vi "Encoder_Open4Encoders.vi"(0 "Rear Left Motor A":T6, 1 "Rear Left Motor B":T6, 2 "Rear Right Motor A":T6, 3 "Rear Right Motor B":T6, 4 "Front Left Motor A":T6, 5 "Front Left Motor B":T6, 6 "Front Right Motor A":T6, 7 "Front Right Motor B":T6, 8 "Front Right Motor Max":dbl, 10 "Front Left Motor Max":dbl, 12 "Rear Right Motor Max":dbl, 14 "Rear Left Motor Max":dbl) -> (21 "RobotEncoderRef Out":T5, 26 "error out":errorcluster)   [LabVIEW 2013]
uses:
  <vilib>/Rock Robotics/SystemInterfaces/DIO/FPGA_DIOChannel.ctl
  <vilib>/Rock Robotics/WPI/Encoder/WPI_EncoderDevRef.ctl
  <vilib>/Rock Robotics/SystemInterfaces/Encoder/FPGA_EncoderIdx.ctl
  <vilib>/Rock Robotics/SystemInterfaces/Counter/FPGA_CounterCtrSystemIndex.ctl
  <vilib>/Rock Robotics/WPI/Encoder/WPI_EncoderType.ctl
  <vilib>/Rock Robotics/WPI/Counter/WPI_CounterDigitalInputToDigitalSource.vi
panel:
  in  "error in (no error)":errorcluster
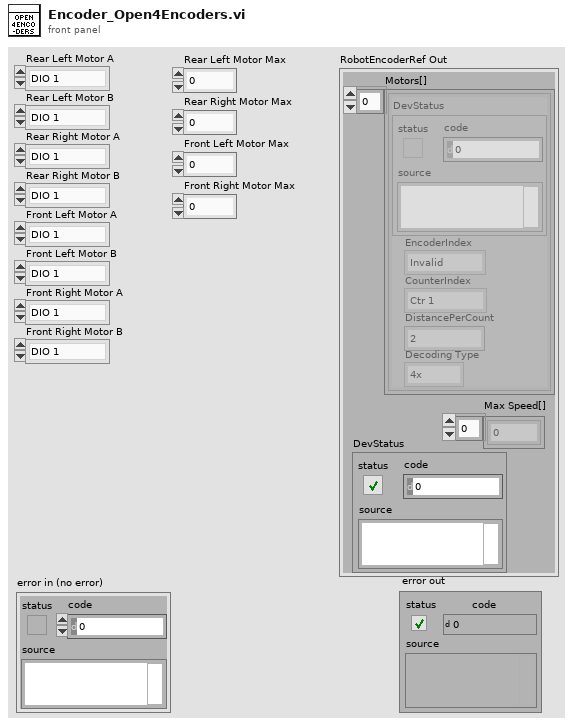
[diagram p1: front panel]
types:
  T1 = typedef "WPI_EncoderDevRef.ctl" = cluster{"DevStatus":errorcluster, "EncoderIndex":T2, "CounterIndex":T3, "DistancePerCount":dbl, "Decoding Type":T4}
  T2 = typedef "FPGA_EncoderIdx.ctl" = enum8{"Enc 0", "Enc 1", "Enc 2", "Enc 3", "Invalid"}
  T3 = typedef "FPGA_CounterCtrSystemIndex.ctl" = enum8{"Ctr 0", "Ctr 1", "Ctr 2", "Ctr 3", "Ctr 4", "Ctr 5", "Ctr 6", "Ctr 7", "Invalid"}
  T4 = typedef "WPI_EncoderType.ctl" = enum16{"1x", "2x", "4x"}
  T5 = cluster{"Motors[]":T1[], "DevStatus":errorcluster, "Max Speed[]":dbl[]}
  T6 = typedef "FPGA_DIOChannel.ctl" = enum8{"DIO 1", "DIO 2", "DIO 3", "DIO 4", "DIO 5", "DIO 6", "DIO 7", "DIO 8", "DIO 9", "DIO 10", "DIO 11", "DIO 12", "DIO 13", "DIO 14", "Invalid"}
  T7 = typedef "WPI_DigitalInputDevRef.ctl" = cluster{"DevStatus":errorcluster, "DIO Channel":T6, "Digital Module":T8}
  T8 = typedef "FPGA_TypedefDigitalModule.ctl" = enum16{"Digital Module 1", "Digital Module 2"}
  T9 = typedef "FPGA_CounterEncoderSourceConvertionLVSourceType.ctl" = cluster{"DevStatus":errorcluster, "AnalogTriggerMode?":bool, "DigitalMode":cluster{"Digital Module":T8, "DIO Channel":T10}, "AnalogTriggerMode":cluster{"AnalogTriggerIndex":T11, "OutputType":T12}}
  T10 = typedef "FPGA_DIODigitalSourceChannel.ctl" = enum8{"DIO 1", "DIO 2", "DIO 3", "DIO 4", "DIO 5", "DIO 6", "DIO 7", "DIO 8", "DIO 9", "DIO 10", "DIO 11", "DIO 12", "DIO 13", "DIO 14", "Disabled"}
  T11 = typedef "FPGA_AnalogTriggerIndex.ctl" = enum8{"Trig 0", "Trig 1", "Trig 2", "Trig 3", "Trig 4", "Trig 5", "Trig 6", "Trig 7", "Invalid"}
  T12 = typedef "FPGA_AnalogTriggerOutType.ctl" = enum16{"InWindow", "TriggerState", "Rising", "Falling"}
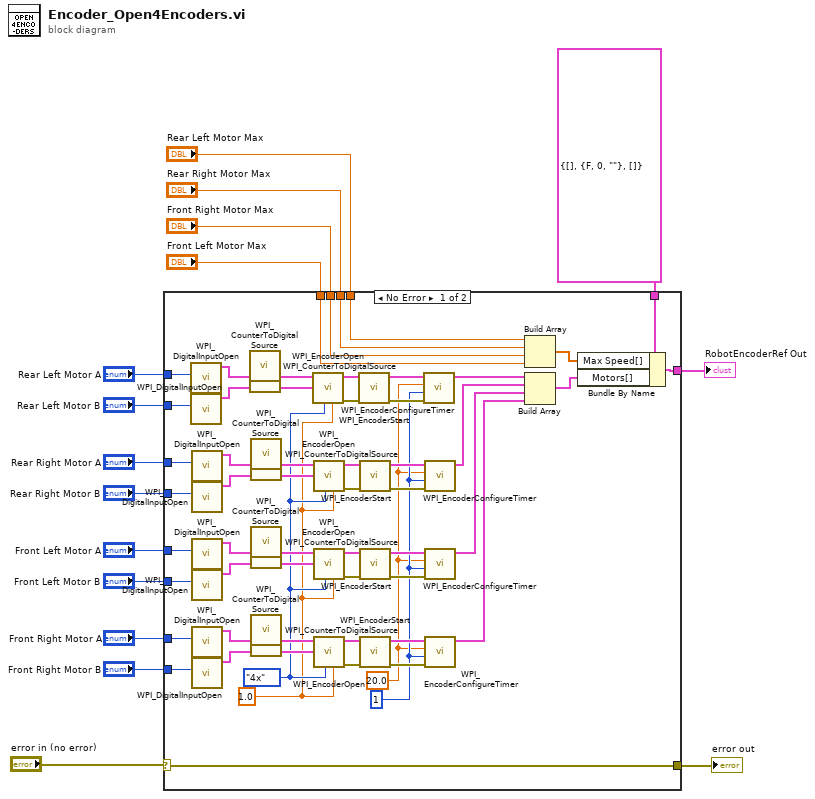
[diagram p0: block diagram]
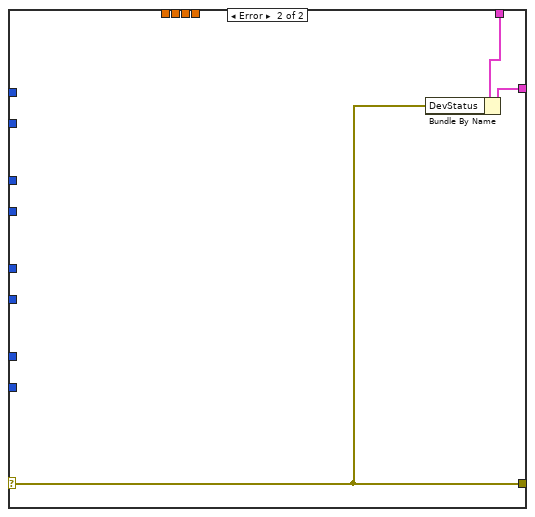
[diagram p2: hidden frame]
diagram:
  n1 = case shown="No Error" "error in (no error)" {
    selector: "error in (no error)" -> [w23 w74]
    tunnel: "Rear Left Motor A" -> [w37 _]
    tunnel: "Rear Left Motor B" -> [w36 _]
    tunnel: "Rear Right Motor A" -> [w35 _]
    tunnel: "Rear Right Motor B" -> [w34 _]
    tunnel: "Front Left Motor A" -> [w33 _]
    tunnel: "Front Left Motor B" -> [w32 _]
    tunnel: "Front Right Motor A" -> [w31 _]
    tunnel: "Front Right Motor B" -> [w30 _]
    tunnel: [w25 w75] -> w7
    tunnel: T5 {"Motors[]"=[], "DevStatus"={"status"=FALSE, "code"=0, "source"=""}, "Max Speed[]"=[]} ("RobotEncoderRef Out") -> [w24 w76]
    tunnel: [w23 w74] -> w8
    tunnel: "Front Left Motor Max" -> [w20 _]
    tunnel: "Front Right Motor Max" -> [w21 _]
    tunnel: "Rear Right Motor Max" -> [w19 _]
    tunnel: "Rear Left Motor Max" -> [w18 _]
    frame No Error {
      w27 = u8 1 ("Number Samples to Average")
      w26 = 20.0 ("Minimum Rate")
      w28 = 1.0 ("DistancePerCount")
      w29 = WPI_EncoderType."4x" ("Decoding Type")
      n2 = call <vilib>:"WPI_DigitalInputOpen.vi"("DIO Channel"=w37) -> ("DigitalInputDevRef"=w66:T7)  [unwired: 9 in, 1 out]
      n3 = call <vilib>:"WPI_DigitalInputOpen.vi"("DIO Channel"=w36) -> ("DigitalInputDevRef"=w67:T7)  [unwired: 9 in, 1 out]
      n4 = call <vilib>:"WPI_DigitalInputOpen.vi"("DIO Channel"=w35) -> ("DigitalInputDevRef"=w58:T7)  [unwired: 9 in, 1 out]
      n5 = call <vilib>:"WPI_DigitalInputOpen.vi"("DIO Channel"=w34) -> ("DigitalInputDevRef"=w59:T7)  [unwired: 9 in, 1 out]
      n6 = call <vilib>:"WPI_DigitalInputOpen.vi"("DIO Channel"=w33) -> ("DigitalInputDevRef"=w50:T7)  [unwired: 9 in, 1 out]
      n7 = call <vilib>:"WPI_DigitalInputOpen.vi"("DIO Channel"=w32) -> ("DigitalInputDevRef"=w51:T7)  [unwired: 9 in, 1 out]
      n8 = call <vilib>:"WPI_DigitalInputOpen.vi"("DIO Channel"=w31) -> ("DigitalInputDevRef"=w42:T7)  [unwired: 9 in, 1 out]
      n9 = call <vilib>:"WPI_DigitalInputOpen.vi"("DIO Channel"=w30) -> ("DigitalInputDevRef"=w43:T7)  [unwired: 9 in, 1 out]
      n10 = call-poly <vilib>:"WPI_CounterToDigitalSource.vi"("DigitalInputDevRef"=w66) -> ("Digital Source"=w69:T9)  [unwired: 6 in]
      n11 = call-poly <vilib>:"WPI_CounterToDigitalSource.vi"("DigitalInputDevRef"=w67) -> ("Digital Source"=w68:T9)  [unwired: 6 in]
      n12 = call-poly <vilib>:"WPI_CounterToDigitalSource.vi"("DigitalInputDevRef"=w58) -> ("Digital Source"=w61:T9)  [unwired: 6 in]
      n13 = call-poly <vilib>:"WPI_CounterToDigitalSource.vi"("DigitalInputDevRef"=w59) -> ("Digital Source"=w60:T9)  [unwired: 6 in]
      n14 = call-poly <vilib>:"WPI_CounterToDigitalSource.vi"("DigitalInputDevRef"=w50) -> ("Digital Source"=w53:T9)  [unwired: 6 in]
      n15 = call-poly <vilib>:"WPI_CounterToDigitalSource.vi"("DigitalInputDevRef"=w51) -> ("Digital Source"=w52:T9)  [unwired: 6 in]
      n16 = call-poly <vilib>:"WPI_CounterToDigitalSource.vi"("DigitalInputDevRef"=w42) -> ("Digital Source"=w45:T9)  [unwired: 6 in]
      n17 = call-poly <vilib>:"WPI_CounterToDigitalSource.vi"("DigitalInputDevRef"=w43) -> ("Digital Source"=w44:T9)  [unwired: 6 in]
      n18 = call <vilib>:"WPI_EncoderOpen.vi"("DistancePerCount"=w28, "Decoding Type"=w29, "BSource"=w68, "ASource"=w69) -> ("error out"=w73:errorcluster, "EncoderDevRef"=w72:T1)  [unwired: 6 in]
      n19 = call <vilib>:"WPI_EncoderOpen.vi"("DistancePerCount"=w28, "Decoding Type"=w29, "BSource"=w60, "ASource"=w61) -> ("error out"=w65:errorcluster, "EncoderDevRef"=w64:T1)  [unwired: 6 in]
      n20 = call <vilib>:"WPI_EncoderOpen.vi"("DistancePerCount"=w28, "Decoding Type"=w29, "BSource"=w52, "ASource"=w53) -> ("error out"=w57:errorcluster, "EncoderDevRef"=w56:T1)  [unwired: 6 in]
      n21 = call <vilib>:"WPI_EncoderOpen.vi"("DistancePerCount"=w28, "Decoding Type"=w29, "BSource"=w44, "ASource"=w45) -> ("error out"=w49:errorcluster, "EncoderDevRef"=w48:T1)  [unwired: 6 in]
      n22 = call <vilib>:"WPI_EncoderStart.vi"("error in (no error)"=w73, "EncoderDevRef"=w72) -> ("error out"=w71:errorcluster, "EncoderDevRef"=w70:T1)  [unwired: 8 in]
      n23 = call <vilib>:"WPI_EncoderStart.vi"("error in (no error)"=w65, "EncoderDevRef"=w64) -> ("error out"=w63:errorcluster, "EncoderDevRef"=w62:T1)  [unwired: 8 in]
      n24 = call <vilib>:"WPI_EncoderStart.vi"("error in (no error)"=w57, "EncoderDevRef"=w56) -> ("error out"=w55:errorcluster, "EncoderDevRef"=w54:T1)  [unwired: 8 in]
      n25 = call <vilib>:"WPI_EncoderStart.vi"("error in (no error)"=w49, "EncoderDevRef"=w48) -> ("error out"=w47:errorcluster, "EncoderDevRef"=w46:T1)  [unwired: 8 in]
      n26 = call <vilib>:"WPI_EncoderConfigureTimer.vi"("error in (no error)"=w71, "Number Samples to Average"=w27, "Minimum Rate"=w26, "EncoderDevRef"=w70) -> ("EncoderDevRef"=w41:T1)  [unwired: 6 in, 1 out]
      n27 = call <vilib>:"WPI_EncoderConfigureTimer.vi"("error in (no error)"=w63, "Number Samples to Average"=w27, "Minimum Rate"=w26, "EncoderDevRef"=w62) -> ("EncoderDevRef"=w40:T1)  [unwired: 6 in, 1 out]
      n28 = call <vilib>:"WPI_EncoderConfigureTimer.vi"("error in (no error)"=w55, "Number Samples to Average"=w27, "Minimum Rate"=w26, "EncoderDevRef"=w54) -> ("EncoderDevRef"=w39:T1)  [unwired: 6 in, 1 out]
      n29 = call <vilib>:"WPI_EncoderConfigureTimer.vi"("error in (no error)"=w47, "Number Samples to Average"=w27, "Minimum Rate"=w26, "EncoderDevRef"=w46) -> ("EncoderDevRef"=w38:T1)  [unwired: 6 in, 1 out]
      n30 = Build Array(w18, w19, w21, w20) -> (w22:dbl[])
      n31 = Build Array(w41, w40, w39, w38) -> (w17:T1[])
      n32 = Bundle By Name(cluster=w24, "Max Speed[]"=w22, "Motors[]"=w17) -> (w25:T5)
    }
    frame Error {
      n33 = Bundle By Name(cluster=w76, "DevStatus"=w74) -> (w75:T5)
    }
  }
  "error out" <- w8
  "RobotEncoderRef Out" <- w7
